vi "EIP Read.vi"() -> (0 "Output":dbl=140152373.0 format="%.3f")   [LabVIEW 2009]
uses:
  MWC Global.vi
panel:
  out "status":bool[](array[boolean])
  out "error out":errorcluster
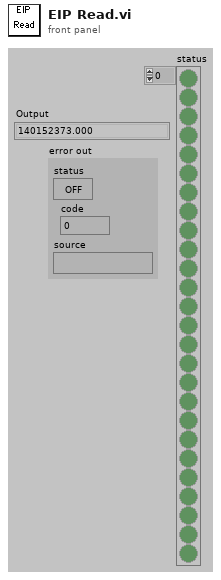
[diagram p1: front panel]
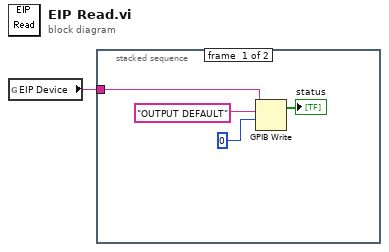
[diagram p0: block diagram]
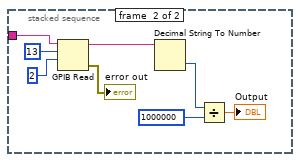
[diagram p2: hidden frame]
diagram:
  n1 = global read "MWC Global.vi" "EIP Device"() -> (w1:string)
  n2 = stacked-sequence {
    tunnel: w1 -> [w4 w12]
    frame #0 {
      n3 = GPIB Write(0:w4, 1:"OUTPUT DEFAULT", 2:i16 0 ("mode (0)")) -> (5:→"status":bool[])  [unwired: 2 in, 1 out]
    }
    frame #1 {
      n4 = GPIB Read(0:w12, 1:13, 2:i16 2 ("mode (0)")) -> (5:w11:string, 7:→"error out":errorcluster)  [unwired: 2 in, 1 out]
      n5 = Decimal String To Number(string=w11) -> (number=w9:i32)  [unwired: 2 in, 1 out]
      n6 = Divide(x=w9, y=1000000) -> (x/y=→"Output":dbl)
    }
  }
